vi "Object detection.vi"() -> ()   [LabVIEW 2018]
uses:
  Underlying VI's/Modified webcam FGV/Webcam AE.ctl
  <vilib>/userdefined/High Color/IMAQdx.ctl
  Underlying VI's/IMAQ Create Reference AE/IMAQ Reference AE.ctl
  Underlying VI's/I2C Master VI/Arduino_Interfacing.ctl
  Underlying VI's/I2C Master VI/I2C_MASTER_WRITE_NEW Type Def.ctl
panel:
  in  "OK Button":bool
  in  "stop":bool
  out "Error out":errorcluster
  out "Object Center Coordinates":cluster{"x":sgl, "y":sgl}
  out "Object detection cluster":T1
  out "Image":T2(plugin-control)
  in  "Mode":enum16{"Ball", "Soap", "Gel", "Pipe", "None"}(ring)
  out "Arduino Data":T3
  out "Position reached?":bool
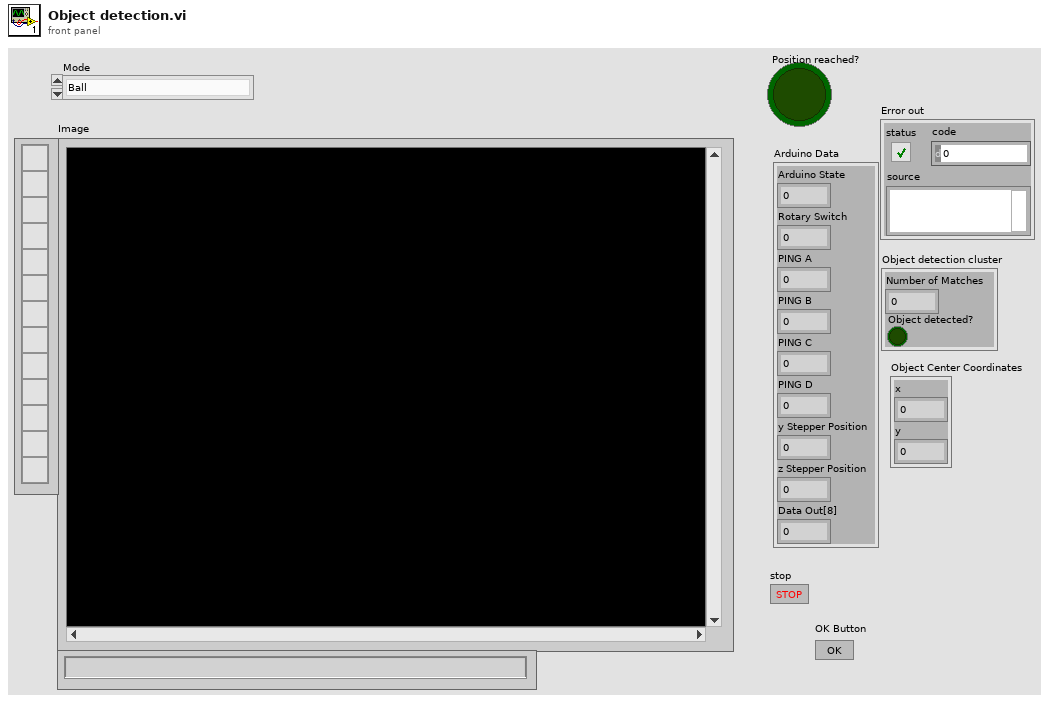
[diagram p1: front panel]
types:
  T1 = cluster{"Number of Matches":i32, "Object detected?":bool}
  T2 = typedef "IMAQ Image.ctl" = refnum<image>
  T3 = cluster{"Arduino State":u8, "Rotary Switch":u8, "PING A":u8, "PING B":u8, "PING C":u8, "PING D":u8, "y Stepper Position":u8, "z Stepper Position":u8, "Data Out[8]":u8}
  T4 = typedef "IMAQ Reference AE.ctl" = enum16{"Initialize AE", "Get IMAQ Reference", "Dispose Processing Buffer"}
  T5 = typedef "Webcam AE.ctl" = enum16{"Initialize Camera", "Open Camera", "Continuous Acquisition", "Close Camera", "Retrieve Image", "Dispose Camera Image Buffer"}
  T6 = typedef "IMAQdx.ctl" = refnum<k21>
  T7 = typedef "I2C_MASTER_WRITE_NEW Type Def.ctl" = enum16{"Ultrasonic sensors", "Stepper origin", "zStepper 13.3k", "zStepper 13k", "zStepper 12k", "zStepper 11k", "zStepper 10k", "zStepper 9k", "zStepper 8k", "zStepper 7k", "zStepper 6k", "zStepper 5k", "zStepper 4k", "zStepper 3k", "zStepper 2k", "zStepper 1k", "zStepper 900", "zStepper 800", "zStepper 700", "zStepper 600", "zStepper 500", "zStepper 400", "zStepper 300", "zStepper 200", "zStepper 100", "zStepper 0", "yStepper control", "Open Claw", "Close Claw", "Soft Reset"}
  T8 = typedef "Arduino_Interfacing.ctl" = enum16{"Initialize", "Write to Arduino", "Read From Arduino"}
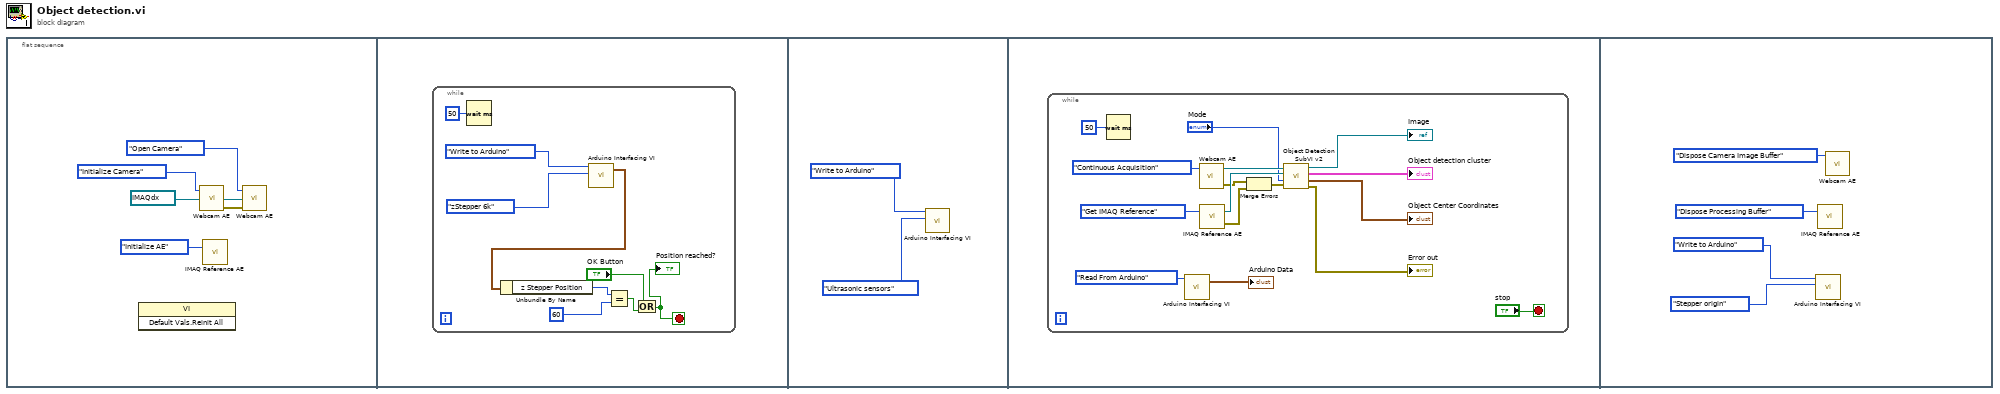
[diagram p0: block diagram]
diagram:
  n1 = flat-sequence {
    frame #0 {
      n2 = invoke class="VI" method="Default Vals.Reinit All"() -> ()  [unwired: 3 in, 3 out]
      n3 = call "Webcam AE.vi"("Session In"=T6 "cam0", "Camera states"=Webcam_AE."Initialize Camera") -> ("error out"=w5:errorcluster, "Session Out"=w6:T6)  [unwired: 1 in, 1 out]
      n4 = call "IMAQ Reference AE.vi"("IMAQ AE States"=IMAQ_Reference_AE."Initialize AE") -> ()  [unwired: 1 in, 2 out]
      n5 = call "Webcam AE.vi"("error in (no error)"=w5, "Session In"=w6, "Camera states"=Webcam_AE."Open Camera") -> ()  [unwired: 3 out]
    }
    frame #1 {
      n6 = while {
        stop <- w7 stop-if-true
        n7 = Wait (ms)(milliseconds to wait=u32 50) -> ()  [unwired: 1 out]
        n8 = call "Arduino Interfacing VI.vi"("Data to Write"=I2C_MASTER_WRITE_NEW_Type_Def."zStepper 6k", "AE Mode"=Arduino_Interfacing."Write to Arduino") -> ("Arduino Data"=w12:T3)  [unwired: 2 in, 1 out]
        n9 = Unbundle By Name(w12) -> ("z Stepper Position"=w10:u8)
        n10 = Equal?(x=w10, y=u8 60) -> (x = y?=w9:bool)
        n11 = Or(x="OK Button", y=w9) -> (x .or. y?=w7:bool)
        "Position reached?" <- w7
      }
    }
    frame #2 {
      n12 = call "Arduino Interfacing VI.vi"("Data to Write"=I2C_MASTER_WRITE_NEW_Type_Def."Ultrasonic sensors", "AE Mode"=Arduino_Interfacing."Write to Arduino") -> ()  [unwired: 2 in, 2 out]
    }
    frame #3 {
      n13 = while {
        stop <- "stop" stop-if-true
        n14 = Wait (ms)(milliseconds to wait=u32 50 ("millisecond timer value")) -> ()  [unwired: 1 out]
        n15 = call "Arduino Interfacing VI.vi"("AE Mode"=Arduino_Interfacing."Read From Arduino") -> ("Arduino Data"=→"Arduino Data":T3)  [unwired: 3 in, 1 out]
        n16 = call "Webcam AE.vi"("Camera states"=Webcam_AE."Continuous Acquisition") -> ("error out"=w22:errorcluster, "Image Out"=w31:T2)  [unwired: 2 in, 1 out]
        n17 = call "IMAQ Reference AE.vi"("IMAQ AE States"=IMAQ_Reference_AE."Get IMAQ Reference") -> ("error out"=w23:errorcluster, "Image Out"=w29:T2)  [unwired: 1 in]
        n18 = Merge Errors(w22, w23) -> (w24:errorcluster)
        n19 = call "Object Detection SubVI v2.vi"("Error In"=w24, "Mode"="Mode", "Image Dest"=w29, "Image in"=w31) -> ("Error out"=→"Error out":errorcluster, "Object Center Coordinates"=→"Object Center Coordinates":cluster{"x":sgl, "y":sgl}, "Object detection cluster"=→"Object detection cluster":T1, "Image Out"=→"Image":T2)
      }
    }
    frame #4 {
      n20 = call "Arduino Interfacing VI.vi"("Data to Write"=I2C_MASTER_WRITE_NEW_Type_Def."Stepper origin", "AE Mode"=Arduino_Interfacing."Write to Arduino") -> ()  [unwired: 2 in, 2 out]
      n21 = call "IMAQ Reference AE.vi"("IMAQ AE States"=IMAQ_Reference_AE."Dispose Processing Buffer") -> ()  [unwired: 1 in, 2 out]
      n22 = call "Webcam AE.vi"("Camera states"=Webcam_AE."Dispose Camera Image Buffer") -> ()  [unwired: 2 in, 3 out]
    }
  }
